vi "Periodic Tasks.vi"(8 "error in":errorcluster) -> ()   [LabVIEW 2019]
doc: "This VI runs in parallel to other tasks. It can contain as many user-defined periodic loops as you need. These can carry out PID or other sorts of timed response."
uses:
  <vilib>/Rock Robotics/WPI/ThirdParty/JAS_Junk/TrajLib/SWERVE_DRIVE_MODULE_STATE.ctl
  <vilib>/Rock Robotics/WPI/ThirdParty/JAS_Junk/TrajLib/ROTATION2D.ctl
  Robot Global Data.vi
  <vilib>/Rock Robotics/Network Tables/NT Write Number.vi
  <vilib>/Rock Robotics/Network Tables/NT Write Boolean.vi
  <vilib>/Rock Robotics/Network Tables/NT Write Numeric Array.vi
  <vilib>/Rock Robotics/Network Tables/NT Write Boolean Array.vi
  Secret_Control_Library_Protected/Secret_Control_Library_Protected.lvlib
  <vilib>/Rock Robotics/WPI/ThirdParty/JAS_Junk/TrajLib/Trajectory_Library.lvlib
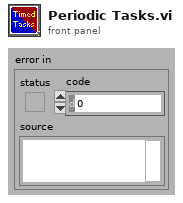
[diagram p1: front panel]
types:
  T1 = typedef "Trajectory_Library.lvlib/SWERVE_DRIVE_MODULE_STATE.ctl" = cluster{"Speed":dbl, "Angle":T2}
  T2 = typedef "Trajectory_Library.lvlib/ROTATION2D.ctl" = cluster{"VALUE":dbl, "COS":dbl, "SIN":dbl}
  T3 = typedef "Trajectory_Library.lvlib/SWERVE_DRIVE_ODOMETRY.ctl" = cluster{"POSE":T4, "GyroOffset":T2, "PreviousAngle":T2, "PrevTime":dbl}
  T4 = typedef "Trajectory_Library.lvlib/POSE2D.ctl" = cluster{"TRANSLATION":T5, "ROTATION":T2}
  T5 = typedef "Trajectory_Library.lvlib/TRANSLATION2D.ctl" = cluster{"X":dbl, "Y":dbl}
  T6 = typedef "WPI_GyroDevRef.ctl" = cluster{"DevStatus":errorcluster, "Analog Channel":T7, "Gain (VoltsPerDegree/Second)":dbl, "Gyro Type":enum16{"Analog", "XRS450"}, "Handle":i32, "SPI Bus":T8, "Device Found":bool, "Sample Rate":dbl, "Calibrate On Open":bool, "Offset":dbl}
  T7 = typedef "FPGA_AIChannel.ctl" = enum8{"AI 0", "AI 1", "AI 2", "AI 3", "AI MXP 0", "AI MXP 1", "AI MXP 2", "AI MXP 3", "Invalid"}
  T8 = typedef "spi_bus.ctl" = enum16{"SPI On-Board, CS0", "SPI On-Board, CS1", "SPI On-Board, CS2", "SPI On-Board, CS3", "SPI MXP", "Invalid"}
  T9 = typedef "SWERVE_MODULE_TYPDEF.ctl" = cluster{"SwervDriveMotor":T10, "SwerveSwerveMotor":T10, "SwerveDriveEnc":T15, "SwerveSwerveEnc":T15}
  T10 = typedef "WPI_MotorControlDeviceRef.ctl" = cluster{"DeviceStatus":errorcluster, "Type":T11, "PWM":cluster{"PWM Channel":T12, "DeadBand":T13}, "CAN":cluster{"Device Number":u8, "SetOutput VI Ref":variant, "GetOutput VI Ref":variant, "Enable VI Ref":variant, "Disable VI Ref":variant, "Data":variant}, "Invert":bool, "DIO PWM":cluster{"PWM \"Enable\" Channel":T12, "DIOChannel":T14, "PWM Rate":dbl}}
  T11 = typedef "WPI_MotorControlType.ctl" = enum16{"PWM", "CAN", "DIO PWM"}
  T12 = typedef "FPGA_DIOPWMChannel.ctl" = enum8{"PWM 0", "PWM 1", "PWM 2", "PWM 3", "PWM 4", "PWM 5", "PWM 6", "PWM 7", "PWM 8", "PWM 9", "PWM MXP 0", "PWM MXP 1", "PWM MXP 2", "PWM MXP 3", "PWM MXP 4", "PWM MXP 5", "PWM MXP 6", "PWM MXP 7", "PWM MXP 8", "PWM MXP 9", "Invalid"}
  T13 = typedef "WPI_PWMDeadband.ctl" = cluster{"Name":string, "maxPositivePwm":i32, "minPositivePwm":i32, "centerPwm":i32, "maxNegativePwm":i32, "minNegativePwm":i32, "angularRange":u16}
  T14 = typedef "FPGA_DIOChannel.ctl" = enum8{"DIO 0", "DIO 1", "DIO 2", "DIO 3", "DIO 4", "DIO 5", "DIO 6", "DIO 7", "DIO 8", "DIO 9", "DIO MXP 0", "DIO MXP 1", "DIO MXP 2", "DIO MXP 3", "DIO MXP 4", "DIO MXP 5", "DIO MXP 6", "DIO MXP 7", "DIO MXP 8", "DIO MXP 9", "DIO MXP 10", "DIO MXP 11", "DIO MXP 12", "DIO MXP 13", "DIO MXP 14", "DIO MXP 15", "SPI Port CS1", "SPI Port CS2", "SPI Port CS3", "SPI Port MISO", "SPI Port MOSI", "Invalid"}
  T15 = typedef "WPI_EncoderDevRef.ctl" = cluster{"DevStatus":errorcluster, "EncoderIndex":T16, "CounterIndex":T17, "DistancePerCount":dbl, "Decoding Type":T18}
  T16 = typedef "FPGA_EncoderIdx.ctl" = enum8{"Enc 0", "Enc 1", "Enc 2", "Enc 3", "Enc 4", "Enc 5", "Enc 6", "Enc 7", "Invalid"}
  T17 = typedef "FPGA_CounterCtrSystemIndex.ctl" = enum8{"Ctr 0", "Ctr 1", "Ctr 2", "Ctr 3", "Ctr 4", "Ctr 5", "Ctr 6", "Ctr 7", "Invalid"}
  T18 = typedef "WPI_EncoderType.ctl" = enum16{"1x", "2x", "4x"}
  T19 = typedef "Trajectory_Library.lvlib/SWERVE_DRIVE_KINEMATICS.ctl" = cluster{"NumModules":i32, "InverseKinematics":T20, "ForwardKinematics":T20, "Modules":T5[], "PrevCoR":T5}
  T20 = typedef "NI_Matrix.lvlib/RealMatrix.ctl" = dbl[][]
  T21 = typedef "Trajectory_Library.lvlib/CHASSIS_SPEEDS.ctl" = cluster{"vX":dbl, "vY":dbl, "vOmega":dbl}
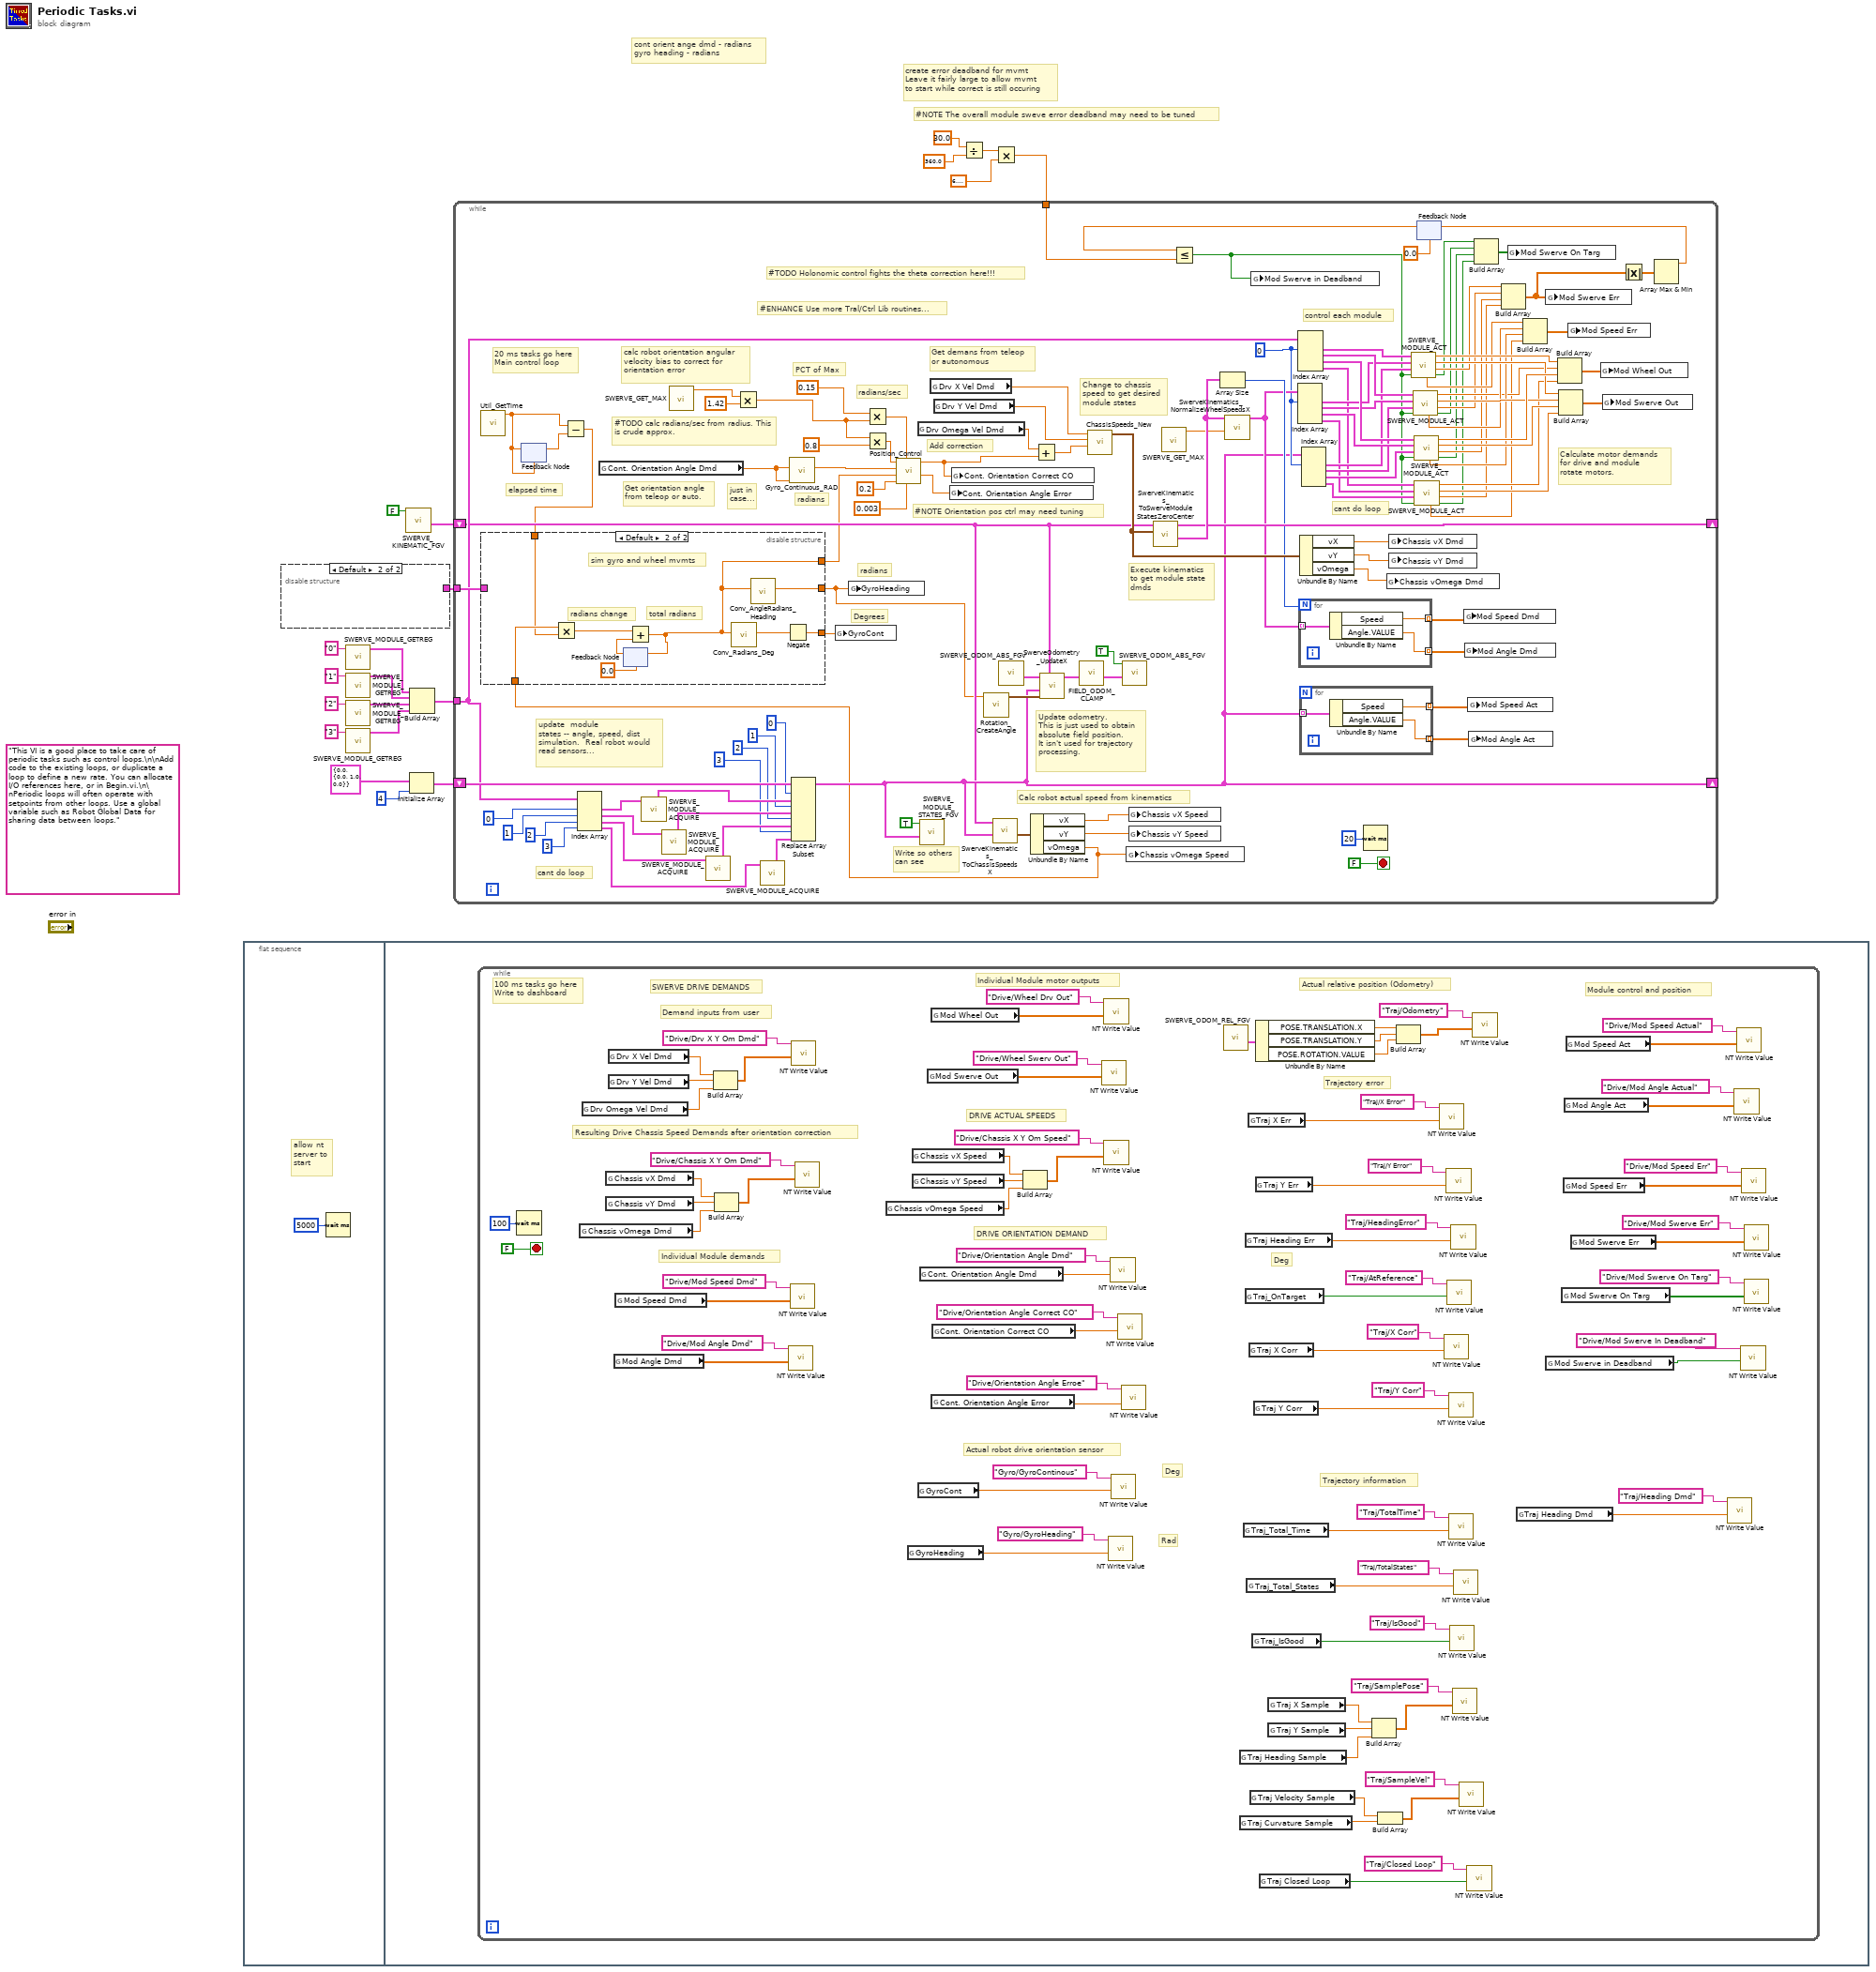
[diagram p0: block diagram]
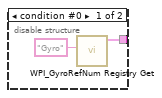
[diagram p2: hidden frame]
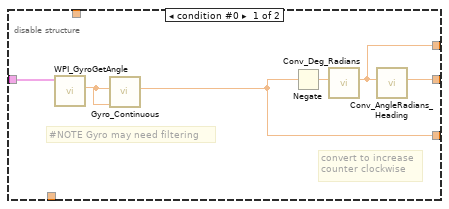
[diagram p3: hidden frame]
diagram:
  (unwired) "This VI is a good place to take care of periodic tasks such as control loops.\n\nAdd code to the existing loops, or duplicate a loop to define a new rate. You can allocate I/O references here, or in Begin.vi.\n\nPeriodic loops will often operate with setpoints from other loops. Use a global variable such as Robot Global Data for sharing data between loops."
  # "cont orient ange dmd - radians\ngyro heading - radians"
  # "#NOTE The overall module sweve error deadband may need to be tuned"
  # "create error deadband for mvmt\nLeave it fairly large to allow mvmt\nto start while correct is still occuring"
  n1 = flat-sequence {
    frame #0 {
      # "allow nt\nserver to \nstart"
      n2 = Wait (ms)(milliseconds to wait=u32 5000) -> ()  [unwired: 1 out]
    }
    frame #1 {
      n3 = while {
        stop <- FALSE stop-if-true
        # "Deg"
        # "Rad"
        # "Deg"
        # "Trajectory information"
        # "Module control and position"
        # "Actual relative position (Odometry)"
        # "Trajectory error"
        # "Actual robot drive orientation sensor"
        # "DRIVE ACTUAL SPEEDS"
        # "DRIVE ORIENTATION DEMAND"
        # "Individual Module motor outputs"
        # "Individual Module demands"
        # "Resulting Drive Chassis Speed Demands after orientation correction"
        # "Demand inputs from user"
        # "SWERVE DRIVE DEMANDS"
        # "100 ms tasks go here\nWrite to dashboard"
        n4 = Wait (ms)(milliseconds to wait=u32 100) -> ()  [unwired: 1 out]
        n5 = global read "Robot Global Data.vi" "Chassis vOmega Dmd"() -> (w80:dbl)
        n6 = global read "Robot Global Data.vi" "Drv Omega Vel Dmd"() -> (w85:dbl)
        n7 = global read "Robot Global Data.vi" "Chassis vX Dmd"() -> (w78:dbl)
        n8 = global read "Robot Global Data.vi" "Chassis vY Dmd"() -> (w79:dbl)
        n9 = global read "Robot Global Data.vi" "Drv X Vel Dmd"() -> (w83:dbl)
        n10 = global read "Robot Global Data.vi" "Drv Y Vel Dmd"() -> (w84:dbl)
        n11 = global read "Robot Global Data.vi" "Mod Angle Dmd"() -> (w73:dbl[])
        n12 = global read "Robot Global Data.vi" "Mod Speed Dmd"() -> (w75:dbl[])
        n13 = Build Array(w83, w84, w85) -> (w82:dbl[])
        n14 = Build Array(w78, w79, w80) -> (w77:dbl[])
        n15 = call-poly <vilib>:"NT Write Value.vi"("Numeric Array"=w73, "Name"="Drive/Mod Angle Dmd") -> ()  [unwired: 9 in, 1 out]
        n16 = call-poly <vilib>:"NT Write Value.vi"("Numeric Array"=w75, "Name"="Drive/Mod Speed Dmd") -> ()  [unwired: 9 in, 1 out]
        n17 = call-poly <vilib>:"NT Write Value.vi"("Numeric Array"=w82, "Name"="Drive/Drv X Y Om Dmd") -> ()  [unwired: 9 in, 1 out]
        n18 = call-poly <vilib>:"NT Write Value.vi"("Numeric Array"=w77, "Name"="Drive/Chassis X Y Om Dmd") -> ()  [unwired: 9 in, 1 out]
        n19 = global read "Robot Global Data.vi" "Chassis vOmega Speed"() -> (w63:dbl)
        n20 = global read "Robot Global Data.vi" "GyroHeading"() -> (w22:dbl)
        n21 = global read "Robot Global Data.vi" "Chassis vX Speed"() -> (w61:dbl)
        n22 = global read "Robot Global Data.vi" "Chassis vY Speed"() -> (w62:dbl)
        n23 = global read "Robot Global Data.vi" "GyroCont"() -> (w102:dbl)
        n24 = global read "Robot Global Data.vi" "Cont. Orientation Angle Dmd"() -> (w86:dbl)
        n25 = global read "Robot Global Data.vi" "Mod Swerve Out"() -> (w65:dbl[])
        n26 = global read "Robot Global Data.vi" "Mod Wheel Out"() -> (w67:dbl[])
        n27 = global read "Robot Global Data.vi" "Cont. Orientation Angle Error"() -> (w57:dbl)
        n28 = global read "Robot Global Data.vi" "Cont. Orientation Correct CO"() -> (w56:dbl)
        n29 = Build Array(w61, w62, w63) -> (w60:dbl[])
        n30 = call-poly <vilib>:"NT Write Value.vi"("Numeric Array"=w65, "Name"="Drive/Wheel Swerv Out") -> ()  [unwired: 9 in, 1 out]
        n31 = call-poly <vilib>:"NT Write Value.vi"("Numeric Array"=w67, "Name"="Drive/Wheel Drv Out") -> ()  [unwired: 9 in, 1 out]
        n32 = call-poly <vilib>:"NT Write Value.vi"("Numeric Array"=w60, "Name"="Drive/Chassis X Y Om Speed") -> ()  [unwired: 9 in, 1 out]
        n33 = call-poly <vilib>:"NT Write Value.vi"("Numeric"=w22, "Name"="Gyro/GyroHeading") -> ()  [unwired: 9 in, 1 out]
        n34 = call-poly <vilib>:"NT Write Value.vi"("Numeric"=w86, "Name"="Drive/Orientation Angle Dmd") -> ()  [unwired: 9 in, 1 out]
        n35 = call-poly <vilib>:"NT Write Value.vi"("Numeric"=w102, "Name"="Gyro/GyroContinous") -> ()  [unwired: 9 in, 1 out]
        n36 = call-poly <vilib>:"NT Write Value.vi"("Numeric"=w56, "Name"="Drive/Orientation Angle Correct CO") -> ()  [unwired: 9 in, 1 out]
        n37 = call-poly <vilib>:"NT Write Value.vi"("Numeric"=w57, "Name"="Drive/Orientation Angle Erroe") -> ()  [unwired: 9 in, 1 out]
        n38 = call "SWERVE_ODOM_REL_FGV.vi"() -> ("out SWERVE_DRIVE_ODOMETRY"=w44:T3)  [unwired: 11 in]
        n39 = global read "Robot Global Data.vi" "Traj Heading Sample"() -> (w39:dbl)
        n40 = global read "Robot Global Data.vi" "Traj Curvature Sample"() -> (w34:dbl)
        n41 = global read "Robot Global Data.vi" "Traj_Total_Time"() -> (w92:dbl)
        n42 = global read "Robot Global Data.vi" "Traj Heading Err"() -> (w96:dbl)
        n43 = global read "Robot Global Data.vi" "Traj_OnTarget"() -> (w94:bool)
        n44 = global read "Robot Global Data.vi" "Traj_Total_States"() -> (w90:dbl)
        n45 = global read "Robot Global Data.vi" "Traj X Err"() -> (w100:dbl)
        n46 = global read "Robot Global Data.vi" "Traj X Corr"() -> (w28:dbl)
        n47 = global read "Robot Global Data.vi" "Traj Velocity Sample"() -> (w33:dbl)
        n48 = global read "Robot Global Data.vi" "Traj_IsGood"() -> (w47:bool)
        n49 = global read "Robot Global Data.vi" "Traj Y Corr"() -> (w26:dbl)
        n50 = global read "Robot Global Data.vi" "Traj Y Err"() -> (w98:dbl)
        n51 = Unbundle By Name(w44) -> ("POSE.TRANSLATION.X"=w43:dbl, "POSE.TRANSLATION.Y"=w42:dbl, "POSE.ROTATION.VALUE"=w41:dbl)
        n52 = global read "Robot Global Data.vi" "Traj Closed Loop"() -> (w31:bool)
        n53 = global read "Robot Global Data.vi" "Traj X Sample"() -> (w37:dbl)
        n54 = global read "Robot Global Data.vi" "Traj Y Sample"() -> (w38:dbl)
        n55 = Build Array(w37, w38, w39) -> (w36:dbl[])
        n56 = Build Array(w33, w34) -> (w32:dbl[])
        n57 = Build Array(w43, w42, w41) -> (w46:dbl[])
        n58 = call-poly <vilib>:"NT Write Value.vi"("Numeric"=w100, "Name"="Traj/X Error") -> ()  [unwired: 9 in, 1 out]
        n59 = call-poly <vilib>:"NT Write Value.vi"("Numeric"=w28, "Name"="Traj/X Corr") -> ()  [unwired: 9 in, 1 out]
        n60 = call-poly <vilib>:"NT Write Value.vi"("Numeric"=w98, "Name"="Traj/Y Error") -> ()  [unwired: 9 in, 1 out]
        n61 = call-poly <vilib>:"NT Write Value.vi"("Boolean"=w94, "Name"="Traj/AtReference") -> ()  [unwired: 9 in, 1 out]
        n62 = call-poly <vilib>:"NT Write Value.vi"("Numeric"=w26, "Name"="Traj/Y Corr") -> ()  [unwired: 9 in, 1 out]
        n63 = call-poly <vilib>:"NT Write Value.vi"("Numeric"=w92, "Name"="Traj/TotalTime") -> ()  [unwired: 9 in, 1 out]
        n64 = call-poly <vilib>:"NT Write Value.vi"("Boolean"=w47, "Name"="Traj/IsGood") -> ()  [unwired: 9 in, 1 out]
        n65 = call-poly <vilib>:"NT Write Value.vi"("Numeric"=w96, "Name"="Traj/HeadingError") -> ()  [unwired: 9 in, 1 out]
        n66 = call-poly <vilib>:"NT Write Value.vi"("Numeric Array"=w36, "Name"="Traj/SamplePose") -> ()  [unwired: 9 in, 1 out]
        n67 = call-poly <vilib>:"NT Write Value.vi"("Numeric"=w90, "Name"="Traj/TotalStates") -> ()  [unwired: 9 in, 1 out]
        n68 = call-poly <vilib>:"NT Write Value.vi"("Numeric Array"=w32, "Name"="Traj/SampleVel") -> ()  [unwired: 9 in, 1 out]
        n69 = call-poly <vilib>:"NT Write Value.vi"("Boolean"=w31, "Name"="Traj/Closed Loop") -> ()  [unwired: 9 in, 1 out]
        n70 = call-poly <vilib>:"NT Write Value.vi"("Numeric Array"=w46, "Name"="Traj/Odometry") -> ()  [unwired: 9 in, 1 out]
        n71 = global read "Robot Global Data.vi" "Traj Heading Dmd"() -> (w24:dbl)
        n72 = global read "Robot Global Data.vi" "Mod Swerve in Deadband"() -> (w49:bool)
        n73 = global read "Robot Global Data.vi" "Mod Swerve On Targ"() -> (w50:bool[])
        n74 = global read "Robot Global Data.vi" "Mod Speed Err"() -> (w52:dbl[])
        n75 = global read "Robot Global Data.vi" "Mod Angle Act"() -> (w69:dbl[])
        n76 = global read "Robot Global Data.vi" "Mod Speed Act"() -> (w71:dbl[])
        n77 = global read "Robot Global Data.vi" "Mod Swerve Err"() -> (w51:dbl[])
        n78 = call-poly <vilib>:"NT Write Value.vi"("Numeric"=w24, "Name"="Traj/Heading Dmd") -> ()  [unwired: 9 in, 1 out]
        n79 = call-poly <vilib>:"NT Write Value.vi"("Numeric Array"=w69, "Name"="Drive/Mod Angle Actual") -> ()  [unwired: 9 in, 1 out]
        n80 = call-poly <vilib>:"NT Write Value.vi"("Numeric Array"=w71, "Name"="Drive/Mod Speed Actual") -> ()  [unwired: 9 in, 1 out]
        n81 = call-poly <vilib>:"NT Write Value.vi"("Boolean"=w49, "Name"="Drive/Mod Swerve In Deadband") -> ()  [unwired: 9 in, 1 out]
        n82 = call-poly <vilib>:"NT Write Value.vi"("Numeric Array"=w52, "Name"="Drive/Mod Speed Err") -> ()  [unwired: 9 in, 1 out]
        n83 = call-poly <vilib>:"NT Write Value.vi"("Numeric Array"=w51, "Name"="Drive/Mod Swerve Err") -> ()  [unwired: 9 in, 1 out]
        n84 = call-poly <vilib>:"NT Write Value.vi"("Boolean Array"=w50, "Name"="Drive/Mod Swerve On Targ") -> ()  [unwired: 9 in, 1 out]
      }
    }
  }
  n85 = disable-structure shown="Default" {
    disable-tunnel: [w106 _] -> w8
    frame condition #0 {
      n86 = call <vilib>:"WPI_GyroRefNum Registry Get.vi"("refnum name"="Gyro") -> ("GyroDevRef"=w106:T6)  [unwired: 9 in, 1 out]
    }
    frame condition #1 (active) {
    }
  }
  n87 = call "SWERVE_MODULE_GETREG.vi"("Suffix"="0" ("NameSuffix")) -> ("Swerve Module TypDef"=w13:T9)  [unwired: 10 in]
  n88 = call "SWERVE_MODULE_GETREG.vi"("Suffix"="1" ("NameSuffix")) -> ("Swerve Module TypDef"=w12:T9)  [unwired: 10 in]
  n89 = call "SWERVE_MODULE_GETREG.vi"("Suffix"="2" ("NameSuffix")) -> ("Swerve Module TypDef"=w11:T9)  [unwired: 10 in]
  n90 = call "SWERVE_MODULE_GETREG.vi"("Suffix"="3" ("NameSuffix")) -> ("Swerve Module TypDef"=w6:T9)  [unwired: 10 in]
  n91 = call "SWERVE_KINEMATIC_FGV.vi"("WRITE"=FALSE) -> ("out SWERVE_DRIVE_KINEMATICS"=w17:T19)  [unwired: 10 in]
  n92 = Initialize Array(T1 {"Speed"=0.0, "Angle"={"VALUE"=0.0, "COS"=1.0, "SIN"=0.0}} ("SWERVE_DRIVE_MODULE_STATE"), 4 ("dimension size")) -> (w18:T1[])
  n93 = Build Array(w13, w12, w11, w6) -> (w10:T9[])
  n94 = Divide(x=30.0, y=360.0) -> (x/y=w3:dbl)
  n95 = Multiply(x=w3, y=6.283185307179586) -> (x*y=w1:dbl)
  n96 = while {
    shift-right: [w161] -> _
    shift-left: w18 -> [w192]
    tunnel: w10 -> [w186]
    shift-right: [w207] -> _
    shift-left: w17 -> [w160]
    tunnel: w8 -> [w204]
    tunnel: w1 -> [w114]
    stop <- FALSE stop-if-true
    w164 = 0 ("index")
    # "#TODO Holonomic control fights the theta correction here!!!"
    # "Calculate motor demands\nfor drive and module \nrotate motors."
    # "Execute kinematics\nto get module state\ndmds"
    # "Get orientation angle\nfrom teleop or auto."
    # "Add correction"
    # "Get demans from teleop\nor autonomous"
    # "Calc robot actual speed from kinematics"
    # "#ENHANCE Use more Tral/Ctrl Lib routines..."
    # "Degrees"
    # "just in\ncase..."
    # "radians"
    # "#TODO calc radians/sec from radius. This is crude approx."
    # "PCT of Max"
    # "Update odometry.\nThis is just used to obtain\nabsolute field position.\nIt isn't used for trajectory\nprocessing."
    # "Write so others\ncan see"
    # "#NOTE Orientation pos ctrl may need tuning"
    # "elapsed time"
    # "cant do loop"
    # "cant do loop"
    # "control each module"
    # "update  module\nstates -- angle, speed, dist\nsimulation.  Real robot would\nread sensors..."
    # "Change to chassis \nspeed to get desired\nmodule states"
    # "radians/sec"
    # "radians"
    # "calc robot orientation angular\nvelocity bias to correct for\norientation error"
    # "20 ms tasks go here\nMain control loop"
    n97 = call <vilib>:"Util_GetTime.vi"() -> ("FPGA_Time_Seconds"=w147:dbl)  [unwired: 10 in, 1 out]
    n98 = feedback #1(w147) -> (w148:dbl)
    n99 = feedback-in #1(w147) -> ()
    n100 = Subtract(x=w147, y=w148) -> (x-y=w146:dbl)
    n101 = Index Array(array=w186, index #1=0 ("index"), index #2=1 ("index"), index #3=2 ("index"), index #4=3 ("index")) -> (element #1=w189:T9, element #2=w188:T9, element #3=w187:T9, element #4=w151:T9)
    n102 = global read "Robot Global Data.vi" "Cont. Orientation Angle Dmd"() -> (w112:dbl)
    n103 = call "SWERVE_MODULE_ACQUIRE.vi"("Swerve Module TypDef"=w189) -> ("Swerve Module State"=w193:T1)  [unwired: 5 in, 5 out]
    n104 = call "SWERVE_MODULE_ACQUIRE.vi"("Swerve Module TypDef"=w188) -> ("Swerve Module State"=w190:T1)  [unwired: 5 in, 5 out]
    n105 = call "SWERVE_GET_MAX.vi"() -> ("Max Wheel Vel (Meter/Sec)"=w123:dbl)  [unwired: 10 in, 1 out]
    n106 = call "SWERVE_MODULE_ACQUIRE.vi"("Swerve Module TypDef"=w187) -> ("Swerve Module State"=w191:T1)  [unwired: 5 in, 5 out]
    n107 = Multiply(x=w123, y=1.42) -> (x*y=w121:dbl)
    n108 = call "SWERVE_MODULE_ACQUIRE.vi"("Swerve Module TypDef"=w151) -> ("Swerve Module State"=w150:T1)  [unwired: 5 in, 5 out]
    n109 = call "Gyro_Continuous_RAD.vi"("GyroInitial"=w112, "GyroInput"=w112) -> ("GyroContinuous"=w111:dbl)  [unwired: 9 in]
    n110 = Replace Array Subset(array=w192, new element #1=w193, index #1=0 ("index"), new element #2=w190, index #2=1 ("index"), new element #3=w191, index #3=2 ("index"), new element #4=w150, index #4=3 ("index")) -> (w161:T1[])
    n111 = Multiply(x=0.15, y=w121) -> (x*y=w215:dbl)
    n112 = Multiply(x=w121, y=0.8) -> (x*y=w145:dbl)
    n113 = global read "Robot Global Data.vi" "Drv Omega Vel Dmd"() -> (w211:dbl)
    n114 = call "SWERVE_MODULE_STATES_FGV.vi"("in Current Module States"=w161, "WRITE"=TRUE) -> ()  [unwired: 9 in, 1 out]
    n115 = global read "Robot Global Data.vi" "Drv X Vel Dmd"() -> (w210:dbl)
    n116 = global read "Robot Global Data.vi" "Drv Y Vel Dmd"() -> (w209:dbl)
    n117 = call <vilib>:"SwerveKinematics_ToChassisSpeedsX.vi"("WheelStates"=w161, "in SWERVE_DRIVE_KINEMATICS"=w160) -> ("Chassis Speed"=w162:T21)  [unwired: 9 in]
    n118 = call "SWERVE_ODOM_ABS_FGV.vi"() -> ("out SWERVE_DRIVE_ODOMETRY"=w218:T3)  [unwired: 11 in]
    n119 = Unbundle By Name(w162) -> ("vX"=w159:dbl, "vY"=w158:dbl, "vOmega"=w157:dbl)
    n120 = disable-structure shown="Default" {
      disable-tunnel: [w231 w238] -> w110
      disable-tunnel: [w229 w237] -> w205
      disable-tunnel: w204 -> [w228 _]
      disable-tunnel: w157 -> [_ w236]
      disable-tunnel: w146 -> [_ w234]
      disable-tunnel: [w227 w233] -> w120
      frame condition #0 {
        # "#NOTE Gyro may need filtering"
        # "convert to increase\ncounter clockwise"
        n121 = call <vilib>:"WPI_GyroGetAngle.vi"("GyroDevRef"=w228) -> ("Angle"=w230:dbl)  [unwired: 6 in, 4 out]
        n122 = call "Gyro_Continuous.vi"("GyroInitial"=w230, "GyroInput"=w230) -> ("GyroContinuous"=w229:dbl)  [unwired: 9 in]
        n123 = Negate(x=w229) -> (-x=w232:dbl)
        n124 = call <vilib>:"Conv_Deg_Radians.vi"("Degress"=w232) -> ("Radians"=w227:dbl)  [unwired: 10 in]
        n125 = call <vilib>:"Conv_AngleRadians_Heading.vi"("Radians"=w227) -> ("Heading"=w231:dbl)  [unwired: 10 in]
      }
      frame condition #1 (active) {
        # "total radians"
        # "radians change"
        # "sim gyro and wheel mvmts"
        n126 = Multiply(x=w236, y=w234) -> (x*y=w239:dbl)
        n127 = feedback #2(0.0) -> (w240:dbl)
        n128 = Add(x=w239, y=w240) -> (x+y=w233:dbl)
        n129 = feedback-in #2(w233) -> ()
        n130 = call <vilib>:"Conv_Radians_Deg.vi"("Radians"=w233) -> ("Degrees"=w235:dbl)  [unwired: 10 in]
        n131 = call <vilib>:"Conv_AngleRadians_Heading.vi"("Radians"=w233) -> ("Heading"=w238:dbl)  [unwired: 10 in]
        n132 = Negate(x=w235) -> (-x=w237:dbl)
      }
    }
    n133 = global write "Robot Global Data.vi" "GyroCont"(w205) -> ()
    n134 = global write "Robot Global Data.vi" "GyroHeading"(w110) -> ()
    n135 = call "Position_Control.vi"("ErrDeadband"=0.003, "MinOutput"=w215, "ErrThreshold"=0.2, "CurrentPosition"=w120, "TargetPosition"=w111, "MaxOutput"=w145) -> ("PositionError"=w139:dbl, "Output"=w140:dbl)  [unwired: 3 in, 1 out]
    n136 = global write "Robot Global Data.vi" "Cont. Orientation Angle Error"(w139) -> ()
    n137 = global write "Robot Global Data.vi" "Cont. Orientation Correct CO"(w140) -> ()
    n138 = call <vilib>:"Rotation_CreateAngle.vi"("Angle"=w110) -> ("ROTATION"=w217:T2)  [unwired: 10 in]
    n139 = Add(x=w211, y=w140) -> (x+y=w163:dbl)
    n140 = call <vilib>:"SwerveOdometry_UpdateX.vi"("SWERVE_DRIVE_KINEMATICS"=w160, "gyroAngle"=w217, "module States"=w161, "in SWERVE_DRIVE_ODOMETRY"=w218) -> ("out SWERVE_DRIVE_ODOMETRY"=w109:T3)  [unwired: 6 in, 1 out]
    n141 = call "FIELD_ODOM_CLAMP.vi"("in SWERVE_DRIVE_ODOMETRY"=w109) -> ("out SWERVE_DRIVE_ODOMETRY"=w108:T3)  [unwired: 10 in]
    n142 = call <vilib>:"ChassisSpeeds_New.vi"("vAngular"=w163, "vY"=w209, "vX"=w210) -> ("CHASSIS"=w202:T21)  [unwired: 8 in]
    n143 = call "SWERVE_ODOM_ABS_FGV.vi"("in SWERVE_DRIVE_ODOMETRY"=w108, "WRITE"=TRUE) -> ()  [unwired: 9 in, 1 out]
    n144 = global write "Robot Global Data.vi" "Chassis vOmega Speed"(w157) -> ()
    n145 = global write "Robot Global Data.vi" "Chassis vX Speed"(w159) -> ()
    n146 = global write "Robot Global Data.vi" "Chassis vY Speed"(w158) -> ()
    n147 = call <vilib>:"SwerveKinematics_ToSwerveModuleStatesZeroCenter.vi"("ChassisSpeeds"=w202, "in SWERVE_DRIVE_KINEMATICS"=w160) -> ("ModuleStates"=w208:T1[], "out SWERVE_DRIVE_KINEMATICS"=w207:T19)  [unwired: 8 in]
    n148 = call "SWERVE_GET_MAX.vi"() -> ("Max Wheel Vel (Meter/Sec)"=w203:dbl)  [unwired: 10 in, 1 out]
    n149 = Array Size(array=w208) -> (size(s)=w198:i32)
    n150 = call <vilib>:"SwerveKinematics_NormalizeWheelSpeedsX.vi"("AttainableMaxSpeed"=w203, "in WheelStates"=w208) -> ("out WheelStates"=w182:T1[])  [unwired: 9 in]
    n151 = Index Array(array=w182, index #1=w164) -> (element #1=w181:T1, element #2=w180:T1, element #3=w179:T1, element #4=w153:T1)  [unwired: 3 in]
    n152 = Index Array(array=w186, index #1=w164) -> (element #1=w185:T9, element #2=w184:T9, element #3=w183:T9, element #4=w154:T9)  [unwired: 3 in]
    n153 = for {
      N: w198 -> [_]
      tunnel: w182 -> [w226] mode=indexing
      tunnel: [w225] -> w197 mode=indexing
      tunnel: [w224] -> w196 mode=indexing
      n154 = Unbundle By Name(w226) -> ("Speed"=w224:dbl, "Angle.VALUE"=w225:dbl)
    }
    n155 = Unbundle By Name(w202) -> ("vX"=w201:dbl, "vY"=w200:dbl, "vOmega"=w199:dbl)
    n156 = for {
      tunnel: w161 -> [w223] mode=indexing
      tunnel: [w222] -> w194 mode=indexing
      tunnel: [w221] -> w195 mode=indexing
      n157 = Unbundle By Name(w223) -> ("Speed"=w221:dbl, "Angle.VALUE"=w222:dbl)
    }
    n158 = Index Array(array=w161, index #1=w164) -> (element #1=w178:T1, element #2=w177:T1, element #3=w176:T1, element #4=w152:T1)  [unwired: 3 in]
    n159 = Wait (ms)(milliseconds to wait=u32 20) -> ()  [unwired: 1 out]
    n160 = global write "Robot Global Data.vi" "Chassis vOmega Dmd"(w199) -> ()
    n161 = global write "Robot Global Data.vi" "Chassis vX Dmd"(w201) -> ()
    n162 = global write "Robot Global Data.vi" "Chassis vY Dmd"(w200) -> ()
    n163 = feedback #3(0.0) -> (w115:dbl)
    n164 = Less Or Equal?(x=w115, y=w114) -> (x <= y?=w113:bool)
    n165 = global write "Robot Global Data.vi" "Mod Swerve in Deadband"(w113) -> ()
    n166 = call "SWERVE_MODULE_ACT.vi"("SwervePosInDeadband"=w113, "Swerve Sense"=w178, "Swerve Dmd"=w181, "Swerve Module TypDef"=w185) -> ("SwerveOnTarget"=w127:bool, "SwervePosError"=w133:dbl, "Swerve Motor Dmd"=w172:dbl, "Wheel Motor Dmd"=w175:dbl, "WheelSpeedErr"=w137:dbl)  [unwired: 3 in]
    n167 = call "SWERVE_MODULE_ACT.vi"("SwervePosInDeadband"=w113, "Swerve Sense"=w177, "Swerve Dmd"=w180, "Swerve Module TypDef"=w184) -> ("SwerveOnTarget"=w126:bool, "SwervePosError"=w132:dbl, "Swerve Motor Dmd"=w171:dbl, "Wheel Motor Dmd"=w134:dbl, "WheelSpeedErr"=w136:dbl)  [unwired: 3 in]
    n168 = call "SWERVE_MODULE_ACT.vi"("SwervePosInDeadband"=w113, "Swerve Sense"=w176, "Swerve Dmd"=w179, "Swerve Module TypDef"=w183) -> ("SwerveOnTarget"=w125:bool, "SwervePosError"=w131:dbl, "Swerve Motor Dmd"=w170:dbl, "Wheel Motor Dmd"=w174:dbl, "WheelSpeedErr"=w135:dbl)  [unwired: 3 in]
    n169 = call "SWERVE_MODULE_ACT.vi"("SwervePosInDeadband"=w113, "Swerve Sense"=w152, "Swerve Dmd"=w153, "Swerve Module TypDef"=w154) -> ("SwerveOnTarget"=w124:bool, "SwervePosError"=w130:dbl, "Swerve Motor Dmd"=w155:dbl, "Wheel Motor Dmd"=w156:dbl, "WheelSpeedErr"=w129:dbl)  [unwired: 3 in]
    n170 = global write "Robot Global Data.vi" "Mod Speed Dmd"(w196) -> ()
    n171 = global write "Robot Global Data.vi" "Mod Angle Dmd"(w197) -> ()
    n172 = global write "Robot Global Data.vi" "Mod Speed Act"(w195) -> ()
    n173 = global write "Robot Global Data.vi" "Mod Angle Act"(w194) -> ()
    n174 = Build Array(w127, w126, w125, w124) -> (w128:bool[])
    n175 = Build Array(w133, w132, w131, w130) -> (w118:dbl[])
    n176 = global write "Robot Global Data.vi" "Mod Swerve On Targ"(w128) -> ()
    n177 = Build Array(w137, w136, w135, w129) -> (w138:dbl[])
    n178 = global write "Robot Global Data.vi" "Mod Swerve Err"(w118) -> ()
    n179 = Build Array(w175, w134, w174, w156) -> (w173:dbl[])
    n180 = Build Array(w172, w171, w170, w155) -> (w169:dbl[])
    n181 = global write "Robot Global Data.vi" "Mod Speed Err"(w138) -> ()
    n182 = global write "Robot Global Data.vi" "Mod Wheel Out"(w173) -> ()
    n183 = global write "Robot Global Data.vi" "Mod Swerve Out"(w169) -> ()
    n184 = Absolute Value(x=w118) -> (abs(x)=w119:dbl[])
    n185 = Array Max & Min(array=w119) -> (max value=w117:dbl)  [unwired: 3 out]
    n186 = feedback-in #3(w117) -> ()
  }
